vi "Sync Ch Set Err Check.vi"(9 "pstErrCheck":T1, 10 "Channel":u8, 11 "devId":i32) -> (1 "pstErrCheck out":T1, 2 "devId out":i32, 3 "function return":i32)   [LabVIEW 2013, in "CHR34XXX.lvlib"]
doc: "DLL BOOL __stdcall CHR34XXX_Sync_Ch_LocalAddr(IN int devId,IN BYTE Channel,IN BYTE LocalAddr); DLL BOOL __stdcall CHR34XXX_Sync_Ch_SetCrc(IN int devId,IN BYTE Channel,IN BYTE CrcVal,IN BYTE CrcOrder); DLL BOOL __stdcall CHR34XXX_Sync_Ch_FrmId(IN int devId,IN BYTE Channel,IN WORD IdCnt,IN WORD IdPos,IN WORD IdOrder); DLL BOOL __stdcall CHR34XXX_Sync_Ch_MonitorEn(IN int devId,IN BYTE Channel,IN BOOL Enabled); DLL BOOL __stdcall CHR34XXX_Sync_Ch_TREdge(IN int devId,IN BYTE Channel,IN BYTE TxEdge,IN BYTE RxEdge); DLL BOOL __stdcall CHR34XXX_Sync_Ch_SetSyncWord(IN int devId,IN BYTE Channel,IN pCHRUART_SYNC_WORD_ST pstSyncWord); DLL BOOL __stdcall CHR34XXX_Sync_Ch_SetErrCheck(IN int devId,IN BYTE Channel,IN pCHRUART_SYNC_ERRCHECK_ST pstErrCheck);"
uses:
  CHR34XXX.lvlib
  CHR34XXX.dll
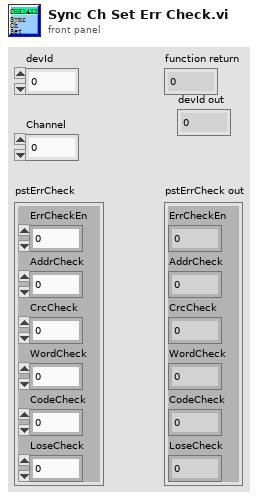
[diagram p1: front panel]
types:
  T1 = cluster{"ErrCheckEn":i32, "AddrCheck":i32, "CrcCheck":i32, "WordCheck":i32, "CodeCheck":i32, "LoseCheck":i32}
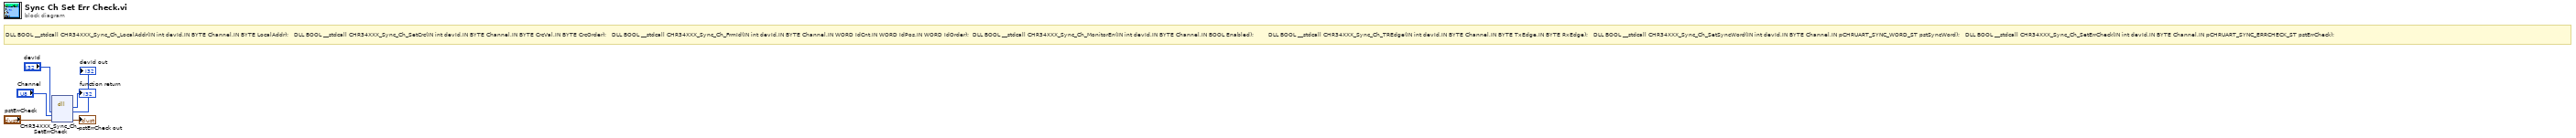
[diagram p0: block diagram]
diagram:
  # "DLL BOOL __stdcall CHR34XXX_Sync_Ch_LocalAddr(IN int devId,IN BYTE Channel,IN BYTE LocalAddr);   DLL BOOL __stdcall CHR34XXX_Sync_Ch_SetCrc(IN int devId,IN BYTE Channel,IN BYTE CrcVal,IN BYTE CrcOrder);   DLL BOOL __stdcall CHR34XXX_Sync_Ch_FrmId(IN int devId,IN BYTE Channel,IN WORD IdCnt,IN WORD IdPos,IN WORD IdOrder);  DLL BOOL __stdcall CHR34XXX_Sync_Ch_MonitorEn(IN int devId,IN BYTE Channel,IN BOOL Enabled);        DLL BOOL __stdcall CHR34XXX_Sync_Ch_TREdge(IN int devId,IN BYTE Channel,IN BYTE TxEdge,IN BYTE RxEdge);   DLL BOOL __stdcall CHR34XXX_Sync_Ch_SetSyncWord(IN int devId,IN BYTE Channel,IN pCHRUART_SYNC_WORD_ST pstSyncWord);   DLL BOOL __stdcall CHR34XXX_Sync_Ch_SetErrCheck(IN int devId,IN BYTE Channel,IN pCHRUART_SYNC_ERRCHECK_ST pstErrCheck);"
  n1 = dll-call lib="C:/Users/Administrator/Desktop/CHR34XXX_lv/lv_lib/CHR34XXX.*" fn="CHR34XXX_Sync_Ch_SetErrCheck"("devId"="devId", "Channel"="Channel", "pstErrCheck"="pstErrCheck") -> ("返回类型"=→"function return":i32, "devId"=→"devId out":i32, "pstErrCheck"=→"pstErrCheck out":T1)  [unwired: 4 in, 2 out]
